vi "Shutdown Event Ref FGV.vi"(7 "Command":T1=enum."Get Event Ref", 8 "error in (no error)":errorcluster) -> (0 "error out":errorcluster, 3 "Shutdown":refnum<user-event>)   [LabVIEW 2018, in "Launcher.lvlib"]
uses:
  Launcher.lvlib
  Shutdown Event FGV Command.ctl
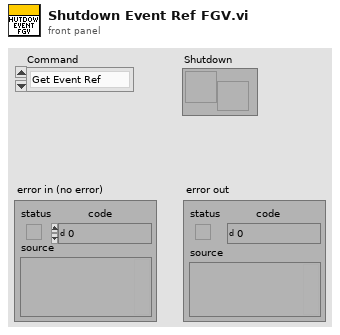
[diagram p1: front panel]
types:
  T1 = typedef "Launcher.lvlib/Shutdown Event FGV Command.ctl" = enum16{"Create Event", "Get Event Ref", "Release Event"}
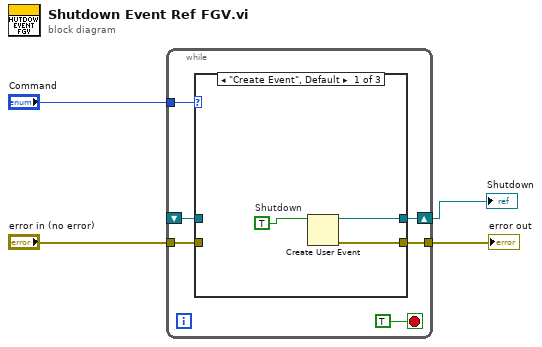
[diagram p0: block diagram]
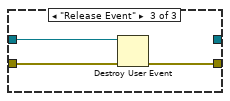
[diagram p3: hidden frame]
diagram:
  n1 = while {
    tunnel: "Command" -> [w9]
    shift-right: [w8] -> w1
    shift-left: _ -> [w7]
    tunnel: [w6] -> w3
    tunnel: "error in (no error)" -> [w5]
    stop <- TRUE stop-if-true
    n2 = case shown="\"Create Event\", Default" w9 {
      tunnel: [w11 w15 _] -> w8
      tunnel: w7 -> [_ w15 w16]
      tunnel: [w13 w14 w17] -> w6
      tunnel: w5 -> [_ w14 w18]
      frame "Create Event", Default {
        w12 = TRUE  # Shutdown
        n3 = Create User Event(user event datatype=w12) -> (user event=w11:refnum<user-event>, error out=w13:errorcluster)  [unwired: 1 in]
      }
      frame "Get Event Ref" {
      }
      frame "Release Event" {
        n4 = Destroy User Event(user event=w16, error in=w18) -> (error out=w17:errorcluster)
      }
    }
  }
  "error out" <- w3
  "Shutdown" <- w1
